vi "GUI_DS-LaserMachiningInputLogger.vi"() -> ()   [LabVIEW 2013]
uses:
  Shared/GUI_Template/GUI_master/tcp_new_data_event.ctl
  Shared/GUI_Template/GUI_master/tcp new data cluster.ctl
panel:
  out "tcp data event":T1
  in  "Refresh Button":bool
  out "XY Graph 4":cluster{timestamp[], dbl[]}(graph)
  in  "Boolean":bool=TRUE caption="Median filter"
  in  "Auto-scale horizontal range":bool caption="Force selected range"
  out "XY Graph 5":cluster{timestamp[], dbl[]}(graph)
  out "XY Graph 3":cluster{timestamp[], dbl[]}(graph)
  in  "Range graph3 (hours) 2":dbl=2.0 caption="Range (hours)"
  in  "MeanCounts::3":dbl caption="LM_Focuscam MeanCounts" min=0.0 max=999999999.0
  in  "MeanCounts::2":dbl caption="LM_Mirrorcam MeanCounts" min=0.0 max=999999999.0
  in  "MeanCounts::4":dbl caption="TS-253a_in MeanCounts" min=0.0 max=999999999.0
  in  "GUIdevice 4":string="TS-253a_in"
  in  "GUIdevice 3":string="LM_Focuscam"
  in  "GUIdevice 2":string="LM_Mirrorcam"
  in  "Number of hours in buffer":dbl=96.0
  out "Current array size":i32
  in  "Range \n(hours)":dbl=48.0
  out "XY Graph 2":cluster{timestamp[], dbl[]}(graph)
  in  "Range\n(hours)":dbl=2.0
  in  "refresh time (ms)":i32=2000
  out "XY Graph":cluster{timestamp[], dbl[]}(graph)
  in  "reading.var 1::1":dbl caption="Regen pulse energy" min=-100000.0 max=100000.0
  in  "stop":bool
  in  "GUIdevice 1":string="DS-LaserFrontEndLogger"
  # "Laser Machining Input logger"
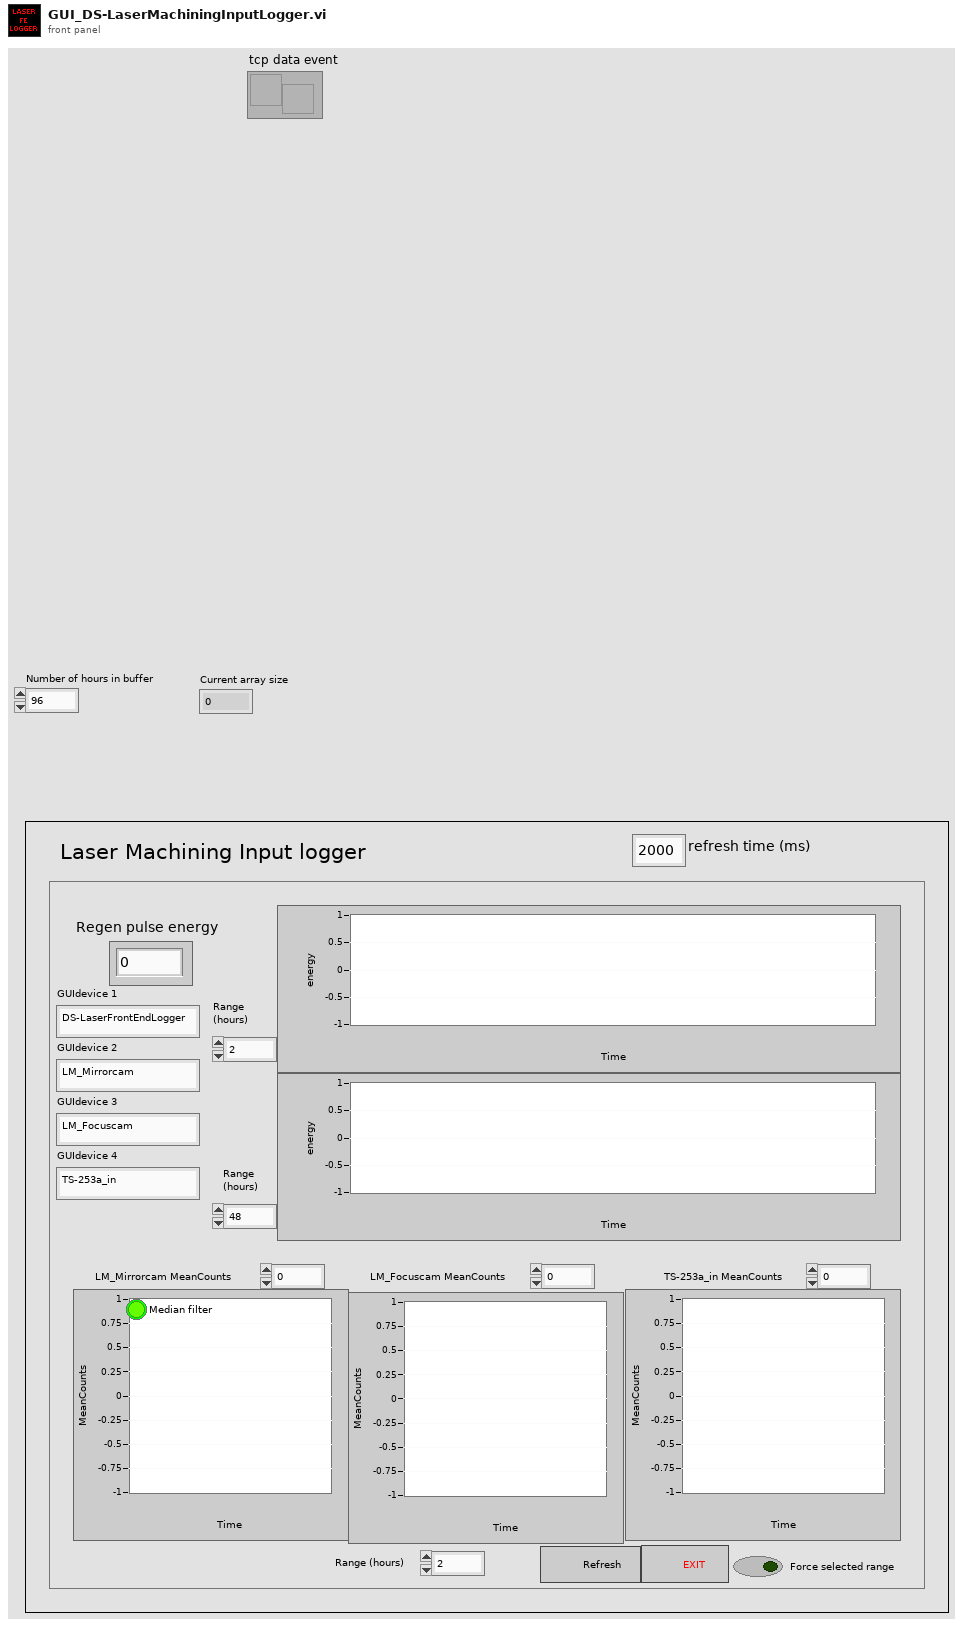
[diagram p1: front panel]
types:
  T1 = typedef "tcp_new_data_event.ctl" = refnum<user-event>
  T2 = enum32{"invalid app kind", "Development System", "Run Time System", "Student Edition", "Embedded LabVIEW", "Evaluation", "Custom"}
  T3 = typedef "tcp new data cluster.ctl" = cluster{"EventEnum":enum16{"new data", "connection status update"}, "Device name":string}
  T4 = enum32{"Invalid", "Standard", "Closed", "Hidden", "Minimized", "Maximized"}
  T5 = cluster{"Core":cluster{"Current VI Reference":refnum<vi>, "Close Panel on Exit?":bool}, "Your Boolean data":bool, "Your string data":string, "SuperGUI":cluster{"STOP queue":refnum<queue>, "SuperGUI ref":refnum<vi>}, "Data":cluster{"Timastamp":dbl[], "variable 1":dbl[], "variable 2":dbl[], "variable 3":dbl[], "variable 4":dbl[], "variable 5":dbl[]}}
  T6 = cluster{"Timastamp":dbl[], "variable 1":dbl[], "variable 2":dbl[], "variable 3":dbl[], "variable 4":dbl[], "variable 5":dbl[]}
  T7 = cluster{"STOP queue":refnum<queue>, "SuperGUI ref":refnum<vi>}
  T8 = cluster{"Current VI Reference":refnum<vi>, "Close Panel on Exit?":bool}
  T9 = cluster{"XY Graph":refnum<vi>, "XY Graph 2":refnum<vi>, "XY Graph 3":refnum<vi>, "XY Graph 4":refnum<vi>, "XY Graph 5":refnum<vi>}
  T10 = cluster{"XY graph":cluster{timestamp[], dbl[]}, "XY graph 2":cluster{timestamp[], dbl[]}, "XY graph 3":cluster{timestamp[], dbl[]}, "XY graph 4":cluster{timestamp[], dbl[]}, "XY graph 5":cluster{timestamp[], dbl[]}}
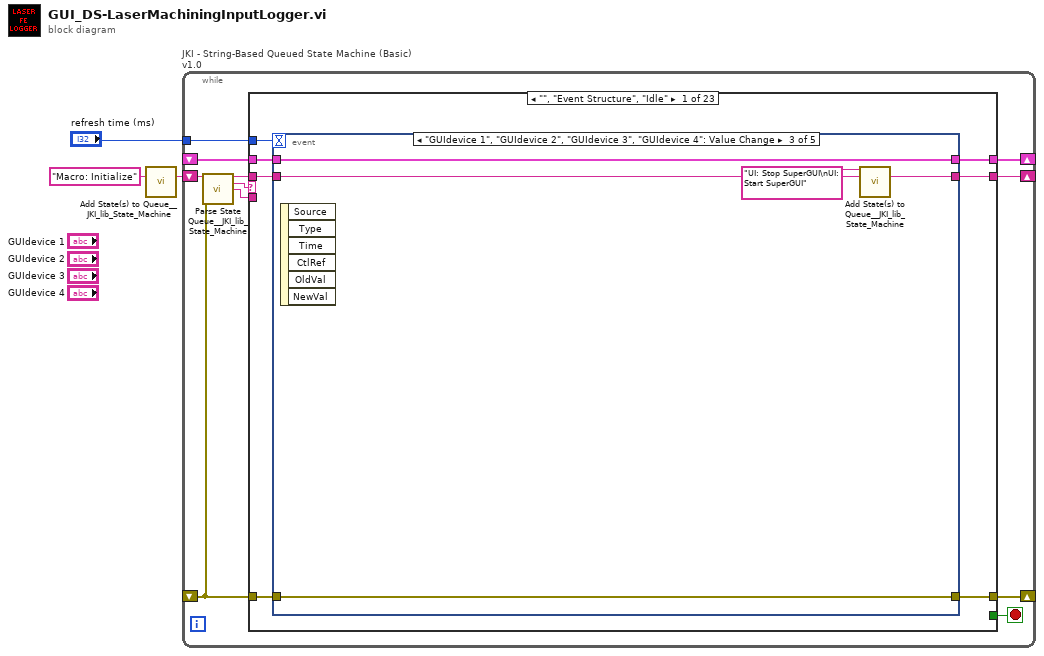
[diagram p0: block diagram]
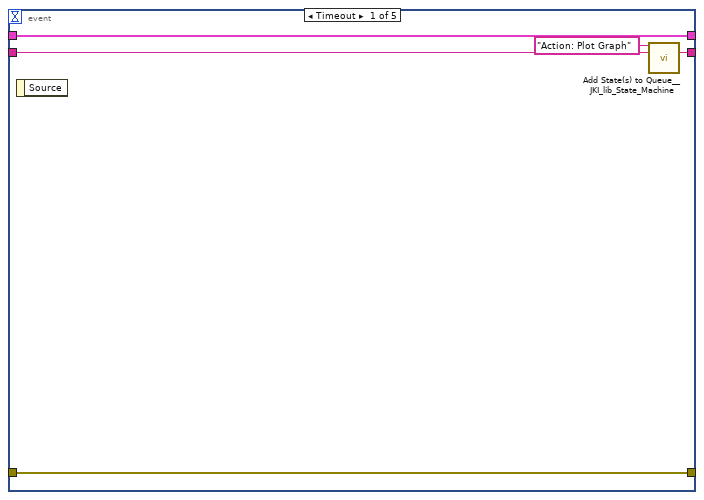
[diagram p2: hidden frame]
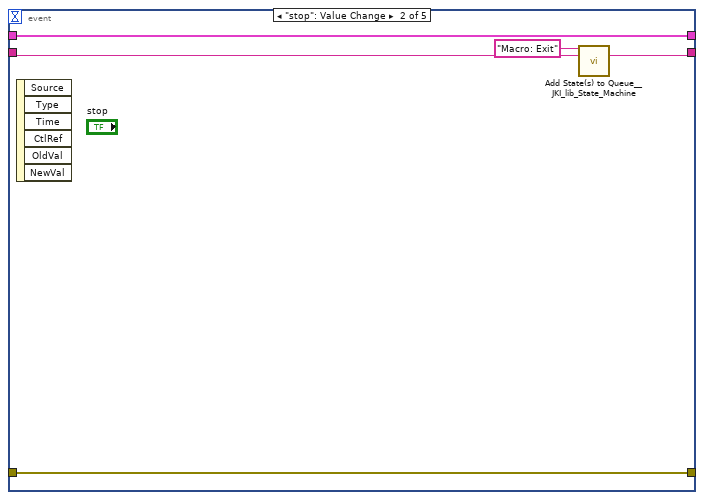
[diagram p3: hidden frame]
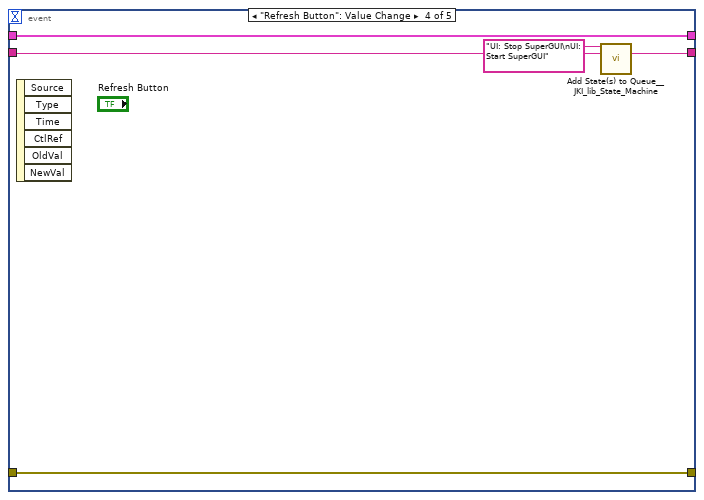
[diagram p4: hidden frame]
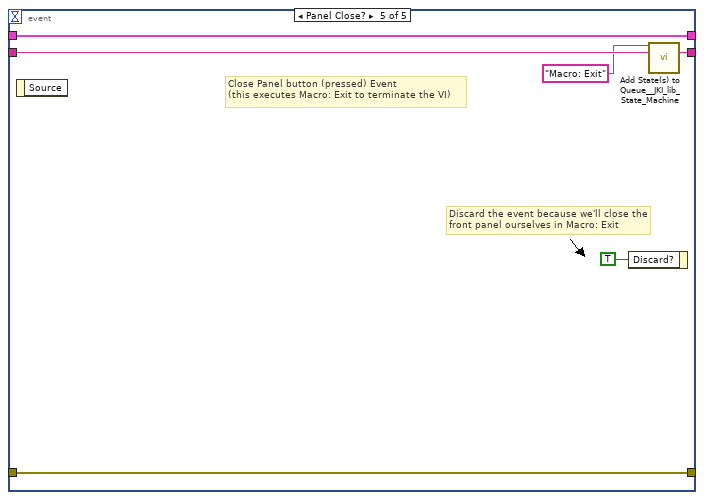
[diagram p5: hidden frame]
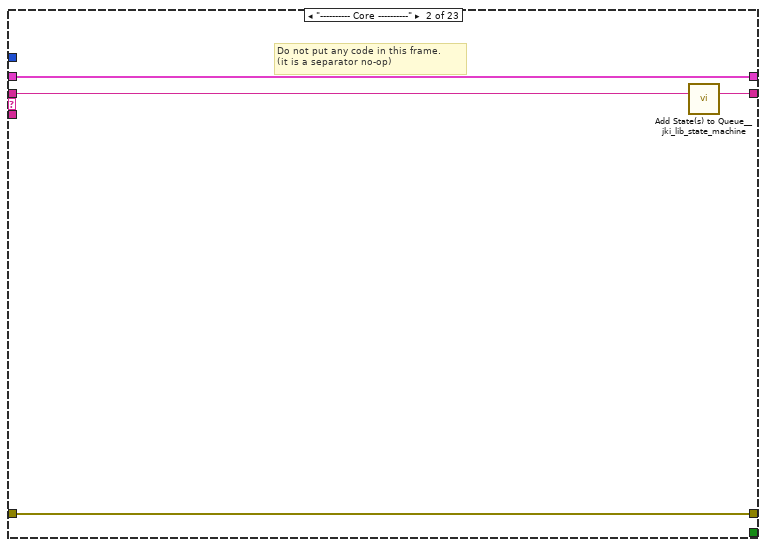
[diagram p6: hidden frame]
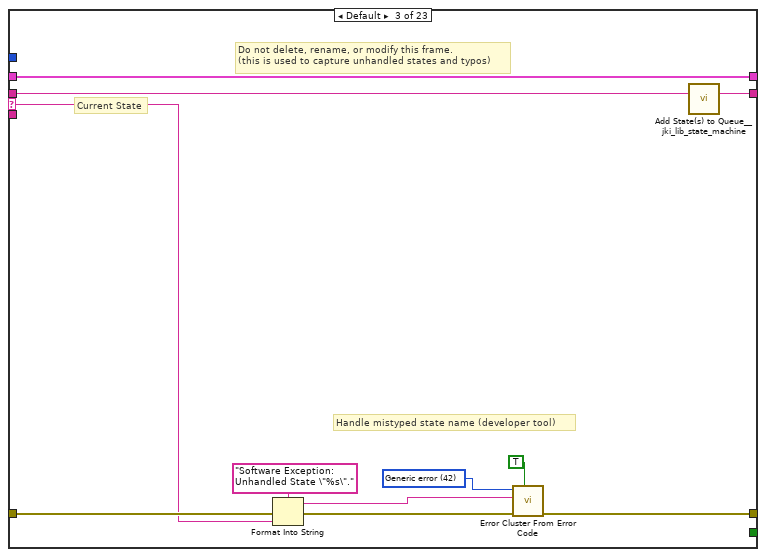
[diagram p7: hidden frame]
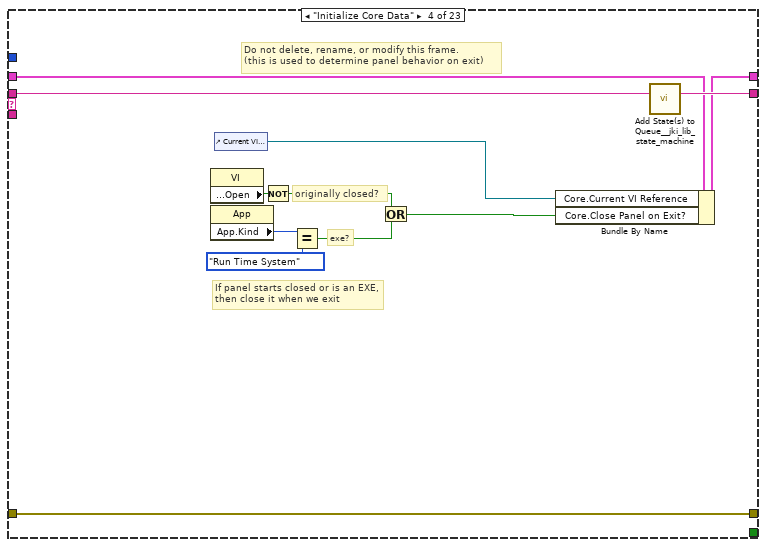
[diagram p8: hidden frame]
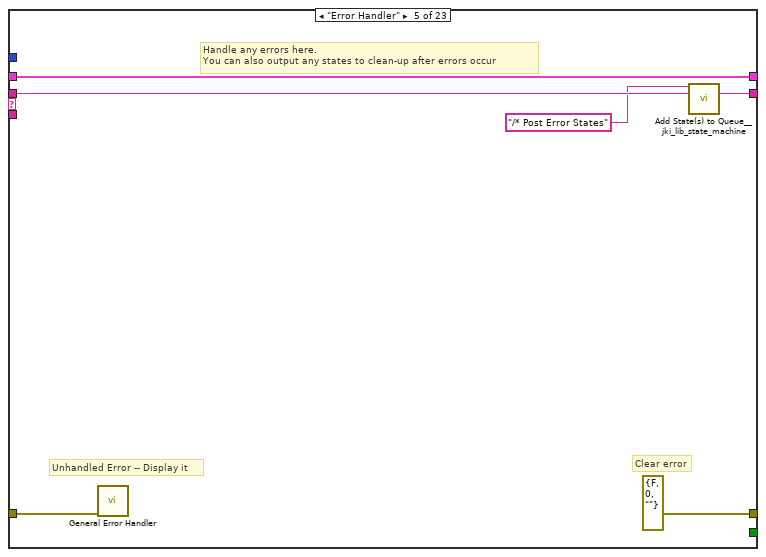
[diagram p9: hidden frame]
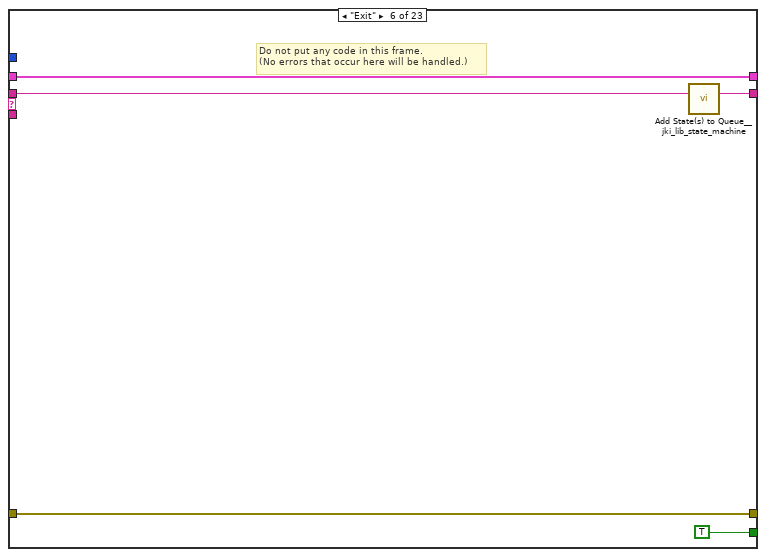
[diagram p10: hidden frame]
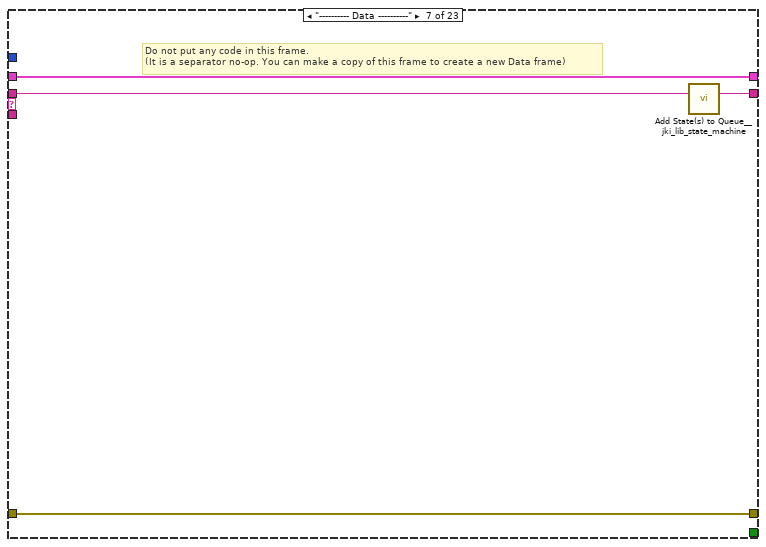
[diagram p11: hidden frame]
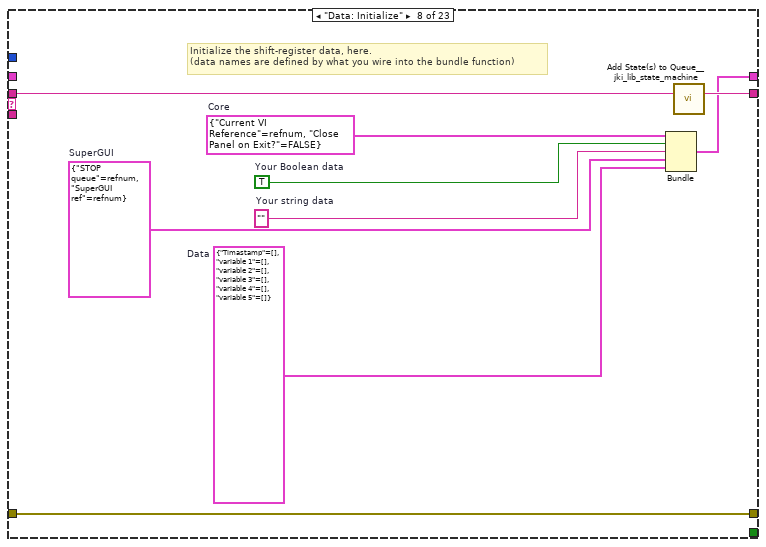
[diagram p12: hidden frame]
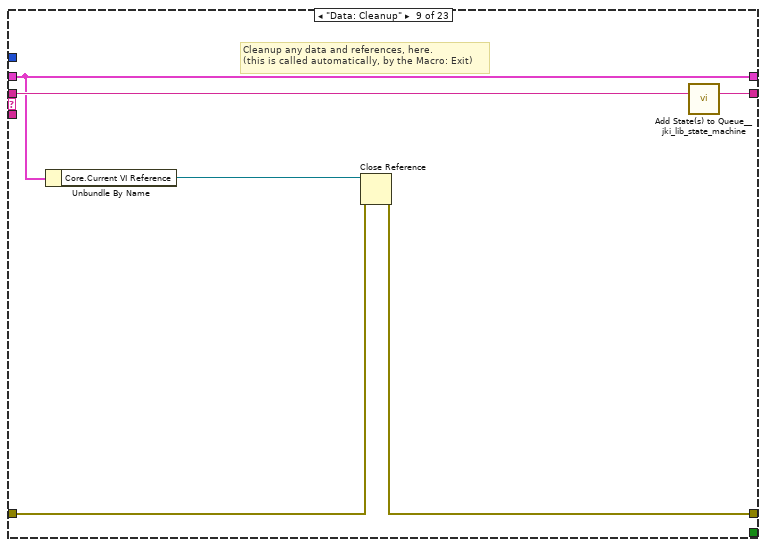
[diagram p13: hidden frame]
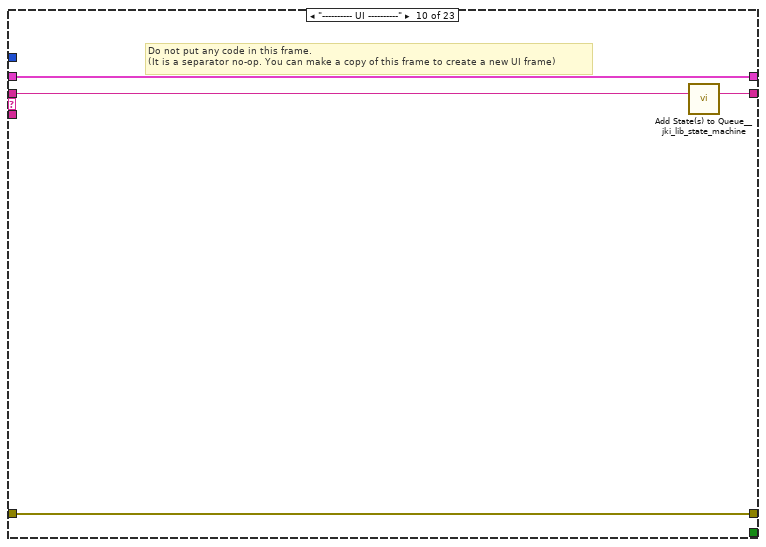
[diagram p14: hidden frame]
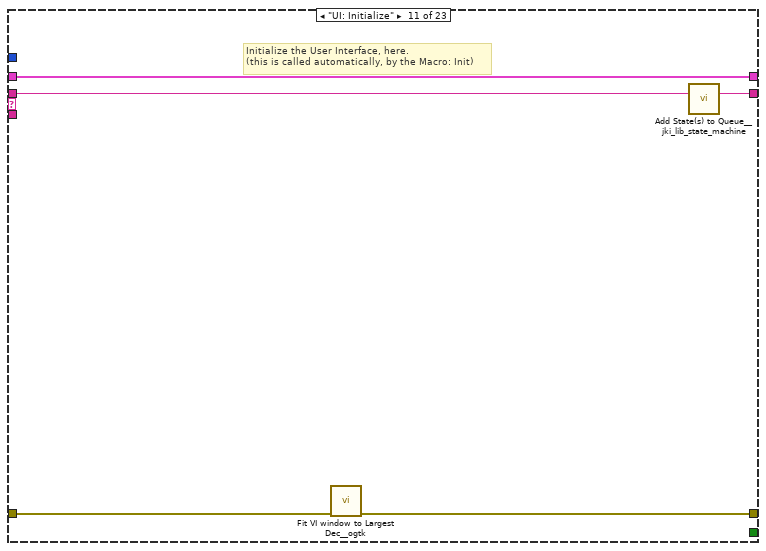
[diagram p15: hidden frame]
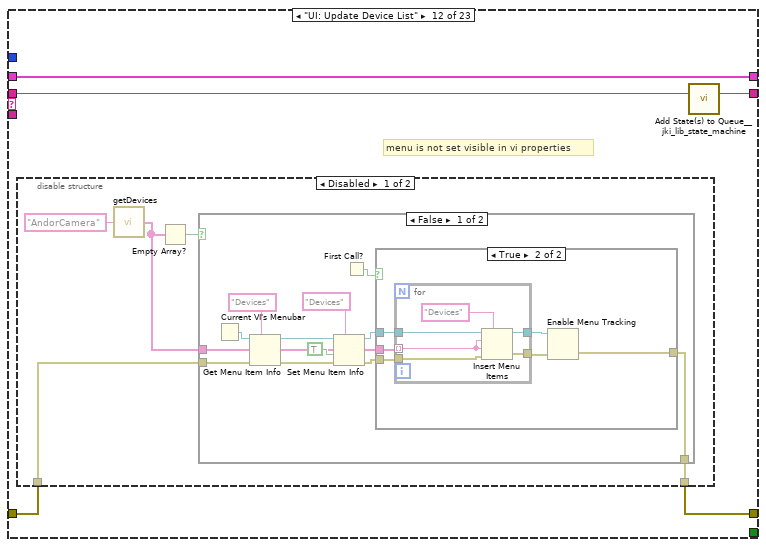
[diagram p16: hidden frame]
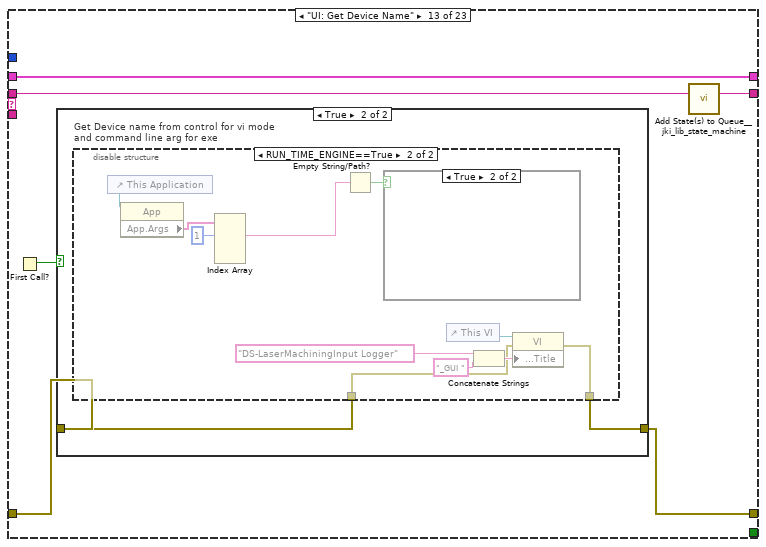
[diagram p20: hidden frame]
diagram:
  n1 = call <vilib>:"Add State(s) to Queue__JKI_lib_State_Machine.vi"("State(s) in (\"\")"="Macro: Initialize") -> ("States Out"=w3:string)  [unwired: 14 in]
  n2 = while "JKI - String-Based Queued State Machine (Basic) v1.0" {
    shift-right: [w7] -> _
    shift-left: _ -> [w6]
    shift-right: [w10] -> _
    shift-left: _ -> [w5]
    shift-right: [w9] -> _
    shift-left: w3 -> [w11]
    tunnel: "refresh time (ms)" -> [w4]
    stop <- w8 stop-if-true
    n3 = call <vilib>:"Parse State Queue__JKI_lib_State_Machine.vi"("State Queue"=w11, "Error In (no error)"=w5) -> ("Remaining States"=w13:string, "Current State"=w14:string, "Arguments"=w12:string)  [unwired: 11 in]
    n4 = case shown="\"\", \"Event Structure\", \"Idle\"" w14 {
      selector: w14 -> [_ _ w52 _ _ _ _ _ _ _ _ _ _ _ _ _ _ _ _ _ _ _ _]
      tunnel: w13 -> [w21 w51 w56 w74 w80 w85 w89 w98 w104 w108 w113 w118 w156 w190 w198 w204 w215 w241 w246 w256 w260 w293 w297]
      tunnel: w12 -> [_ _ _ _ _ _ _ _ _ _ _ _ _ _ _ w199 w209 _ _ _ _ _ _]
      tunnel: w6 -> [w19 w48 w54 w65 w77 w83 w86 _ w99 w105 w111 w116 w154 w181 w193 w202 w211 w238 w243 w253 w257 w269 w294]
      tunnel: [w18 w49 w58 w71 errorcluster {"status"=FALSE, "code"=0, "source"=""} ("error out") w82 w87 w95 w100 w106 w109 w114 w151 w174 w191 w200 w212 w239 w244 w254 w258 w291 w295] -> w10
      tunnel: w5 -> [w17 w49 w57 w71 w76 w82 w87 w95 w101 w106 w110 w115 w152 w175 w192 w201 w213 w239 w244 w254 w258 w291 w295]
      tunnel: [w20 w50 w55 w73 w79 w84 w88 w97 w103 w107 w112 w117 w155 w189 w197 w203 w214 w240 w245 w255 w259 w292 w296] -> w9
      tunnel: [_ _ _ _ _ TRUE _ _ _ _ _ _ _ _ _ _ _ _ _ _ _ _ _] -> w8
      tunnel: [w16 w48 w54 w72 w77 w83 w86 w96 w99 w105 w111 w116 w154 w180 w193 w202 w211 w238 w243 w253 w257 w268 w294] -> w7
      tunnel: w4 -> [w15 _ _ _ _ _ _ _ _ _ _ _ _ _ _ _ _ _ _ _ _ w283 _]
      frame "", "Event Structure", "Idle" {
        n5 = event shown="[2] \"GUIdevice 1\", \"GUIdevice 2\", \"GUIdevice 3\", \"GUIdevice 4\": Value Change" {
          selector: _ -> [_ _ _ _ _]
          dyn-events: _ -> [_ _ _ _ _]
          timeout: w15 -> [_ _ _ _ _]
          tunnel: w21 -> [w26 w29 w35 w39 w47]
          tunnel: [w25 w28 w34 w38 w46] -> w20
          tunnel: w19 -> [w23 w31 w36 w41 w44]
          tunnel: [w24 w30 w32 w40 w45] -> w18
          tunnel: w17 -> [w24 w30 w32 w40 w45]
          tunnel: [w23 w31 w36 w41 w44] -> w16
          event Timeout {
            n6 = event-data() -> ()  [unwired: 1 in, 1 out]
            n7 = call <vilib>:"Add State(s) to Queue__JKI_lib_State_Machine.vi"("State(s) in Front (\"\")"="Action: Plot Graph" ("State(s) in Front (\"\")"), "State(s) in (\"\")"=w26) -> ("States Out"=w25:string)  [unwired: 13 in]
          }
          event "stop": Value Change {
            n8 = event-data() -> ()  [unwired: 1 in, 6 out]
            n9 = call <vilib>:"Add State(s) to Queue__JKI_lib_State_Machine.vi"("State(s) in Front (\"\")"="Macro: Exit", "State(s) in (\"\")"=w29) -> ("States Out"=w28:string)  [unwired: 13 in]
          }
          event "GUIdevice 1", "GUIdevice 2", "GUIdevice 3", "GUIdevice 4": Value Change {
            n10 = event-data() -> ()  [unwired: 1 in, 6 out]
            n11 = call <vilib>:"Add State(s) to Queue__JKI_lib_State_Machine.vi"("State(s) in Front (\"\")"="UI: Stop SuperGUI\nUI: Start SuperGUI", "State(s) in (\"\")"=w35) -> ("States Out"=w34:string)  [unwired: 13 in]
          }
          event "Refresh Button": Value Change {
            n12 = event-data() -> ()  [unwired: 1 in, 6 out]
            n13 = call <vilib>:"Add State(s) to Queue__JKI_lib_State_Machine.vi"("State(s) in Front (\"\")"="UI: Stop SuperGUI\nUI: Start SuperGUI", "State(s) in (\"\")"=w39) -> ("States Out"=w38:string)  [unwired: 13 in]
          }
          event Panel Close? {
            # "Discard the event because we'll close the front panel ourselves in Macro: Exit"
            # "Close Panel button (pressed) Event\n(this executes Macro: Exit to terminate the VI)"
            n14 = event-data() -> ()  [unwired: 1 in, 1 out]
            n15 = event-data("Discard?"=TRUE) -> ()  [unwired: 1 in, 1 out]
            n16 = call <vilib>:"Add State(s) to Queue__JKI_lib_State_Machine.vi"("State(s) in Front (\"\")"="Macro: Exit", "State(s) in (\"\")"=w47) -> ("States Out"=w46:string)  [unwired: 13 in]
          }
        }
      }
      frame "---------- Core ----------" {
        # "Do not put any code in this frame.\n(it is a separator no-op)"
        n17 = call <vilib>:"Add State(s) to Queue__jki_lib_state_machine.vi"("State(s) in (\"\")"=w51) -> ("States Out"=w50:string)  [unwired: 14 in]
      }
      frame Default {
        w61 = 42 items=["No error", "Argument error", "Memory is full", "Out of zone", "End of file", "File already open", "Generic file I/O error", "File not found", "File permission error", "Disk is full", "Duplicate path", "Too many files open", "System feature not enabled", "Resource file not found", "Cannot add resource", "Resource not found", "Image not found", "Image memory error", "Pen does not exist", "Config type invalid", "Config token not found", "Config parse error", "Config memory error", "Bad external code format", "Bad external code offset", "External code not present", "Null window", "Destroy window error", "Null menu", "Print aborted", "Bad print record", "Print driver error", "Windows error during printing", "Memory error during printing", "Print dialog error", "Generic print error", "Invalid device refnum", "Device not found", "Device parameter error", "Device unit error", "Cannot open device", "Device call aborted", "Generic error", "Cancelled by user", "Object ID too low", "Object ID too high", "Object not in heap", "Unknown heap", "Unknown object (invalid DefProc)", "Unknown object (DefProc not in table)", "Message out of range", "Invalid (null) method", "Unknown message", "Manager call not supported", "Bad address", "Network operation in progress", "Network operation timed out", "Connection is busy", "Network attribute not supported", "Network error", "Address in use", "System out of memory", "Connection aborted", "Connection refused", "Not connected", "Already connected", "Connection closed", "Initialization error (interapplication manager)", "Bad occurrence", "Wait on unbound occurrence handler", "Occurrence queue overflow", "Datalog type conflict", "Unused", "Unrecognized type (interapplication manager)", "Memory corrupt", "Failed to make temporary DLL", "Old CIN version", "Drag socket not found", "Failed to load drop-object", "Failed to register OLE object", "Failed to release OLE object", "Format specifier type mismatch", "Unknown format specifier", "Too few format specifiers", "Too many format specifiers", "Scan failed", "Newer CIN version", "Error converting to variant", "Runtime menu error", "Password tampered", "Variant attribute not found", "Incompatible variant data type", "Event data is not available", "Event Store is not present", "Occurrence is not found", "Event Queue is not created", "Event info is not available", "Refnum passed is NULL", "Error retrieving Class GUID", "Error retrieving CoClass GUID", "Error retrieving TypeLib GUID.", "Bad built application magic bytes.", "Specific driver is different from the specific driver associated with the Logical Name.", "There is no session opened to the class driver.", "Max Error", "MAX - Error with config objects", "MAX - Error loading configuration", "MAX - Group not supported"]
        # "Current State"
        # "Do not delete, rename, or modify this frame.\n(this is used to capture unhandled states and typos)"
        # "Handle mistyped state name (developer tool)"
        n18 = Format Into String(format string="Software Exception: Unhandled State \"%s\"." ("message"), error in=w57, w52) -> (resulting string=w60:string, error out=w59:errorcluster)  [unwired: 1 in]
        n19 = call <vilib>:"Error Cluster From Error Code.vi"("show call chain? (False)"=TRUE, "error in (no error)"=w59, "error message (\"\")"=w60, "error code (0)"=w61) -> ("error out"=w58:errorcluster)  [unwired: 5 in]
        n20 = call <vilib>:"Add State(s) to Queue__jki_lib_state_machine.vi"("State(s) in (\"\")"=w56) -> ("States Out"=w55:string)  [unwired: 14 in]
      }
      frame "Initialize Core Data" {
        # "Do not delete, rename, or modify this frame.\n(this is used to determine panel behavior on exit)"
        # "originally closed?"
        # "exe?"
        # "If panel starts closed or is an EXE, then close it when we exit"
        n21 = property class="VI"() -> ("Front Panel.Open"=w70:bool)  [unwired: 2 in, 2 out]
        n22 = property class="App"() -> ("App.Kind"=w69:T2)  [unwired: 2 in, 2 out]
        n23 = control-ref of="Current VI Reference"() -> (w63:refnum<vi>)
        n24 = Not(x=w70) -> (.not. x?=w67:bool)
        n25 = Equal?(x=w69, y=T2."Run Time System" ("Application:Kind")) -> (x = y?=w66:bool)
        n26 = Or(x=w67, y=w66) -> (x .or. y?=w64:bool)
        n27 = Bundle By Name(cluster=w65, "Core.Current VI Reference"=w63, "Core.Close Panel on Exit?"=w64) -> (w72:T5)
        n28 = call <vilib>:"Add State(s) to Queue__jki_lib_state_machine.vi"("State(s) in (\"\")"=w74) -> ("States Out"=w73:string)  [unwired: 14 in]
      }
      frame "Error Handler" {
        # "Unhandled Error -- Display it"
        # "Handle any errors here.\nYou can also output any states to clean-up after errors occur"
        # "Clear error"
        n29 = call <vilib>:"General Error Handler.vi"("error in (no error)"=w76) -> ()  [unwired: 10 in, 5 out]
        n30 = call <vilib>:"Add State(s) to Queue__jki_lib_state_machine.vi"("State(s) in Front (\"\")"="/* Post Error States", "State(s) in (\"\")"=w80) -> ("States Out"=w79:string)  [unwired: 13 in]
      }
      frame "Exit" {
        # "Do not put any code in this frame.\n(No errors that occur here will be handled.)"
        n31 = call <vilib>:"Add State(s) to Queue__jki_lib_state_machine.vi"("State(s) in (\"\")"=w85) -> ("States Out"=w84:string)  [unwired: 14 in]
      }
      frame "---------- Data ----------" {
        # "Do not put any code in this frame.\n(It is a separator no-op. You can make a copy of this frame to create a new Data frame)"
        n32 = call <vilib>:"Add State(s) to Queue__jki_lib_state_machine.vi"("State(s) in (\"\")"=w89) -> ("States Out"=w88:string)  [unwired: 14 in]
      }
      frame "Data: Initialize" {
        w90 = T6 {"Timastamp"=[], "variable 1"=[], "variable 2"=[], "variable 3"=[], "variable 4"=[], "variable 5"=[]}  # Data
        w91 = T7 {"STOP queue"=refnum, "SuperGUI ref"=refnum}  # SuperGUI
        w92 = T8 {"Current VI Reference"=refnum, "Close Panel on Exit?"=FALSE}  # Core
        w94 = TRUE  # Your Boolean data
        w93 = ""  # Your string data
        # "Initialize the shift-register data, here.\n(data names are defined by what you wire into the bundle function)"
        n33 = Bundle("Core"=w92, "Your Boolean data"=w94, "Your string data"=w93, "SuperGUI"=w91, "Data"=w90) -> (w96:T5)  [unwired: 1 in]
        n34 = call <vilib>:"Add State(s) to Queue__jki_lib_state_machine.vi"("State(s) in (\"\")"=w98) -> ("States Out"=w97:string)  [unwired: 14 in]
      }
      frame "Data: Cleanup" {
        # "Cleanup any data and references, here.\n(this is called automatically, by the Macro: Exit)"
        n35 = Unbundle By Name(w99) -> ("Core.Current VI Reference"=w102:refnum<vi>)
        n36 = Close Reference(reference=w102, error in (no error)=w101) -> (error out=w100:errorcluster)
        n37 = call <vilib>:"Add State(s) to Queue__jki_lib_state_machine.vi"("State(s) in (\"\")"=w104) -> ("States Out"=w103:string)  [unwired: 14 in]
      }
      frame "---------- UI ----------" {
        # "Do not put any code in this frame.\n(It is a separator no-op. You can make a copy of this frame to create a new UI frame)"
        n38 = call <vilib>:"Add State(s) to Queue__jki_lib_state_machine.vi"("State(s) in (\"\")"=w108) -> ("States Out"=w107:string)  [unwired: 14 in]
      }
      frame "UI: Initialize" {
        # "Initialize the User Interface, here.\n(this is called automatically, by the Macro: Init)"
        n39 = call <userlib>:"Fit VI window to Largest Dec__ogtk.vi"("error in (no error)"=w110) -> ("error out"=w109:errorcluster)  [unwired: 5 in, 1 out]
        n40 = call <vilib>:"Add State(s) to Queue__jki_lib_state_machine.vi"("State(s) in (\"\")"=w113) -> ("States Out"=w112:string)  [unwired: 14 in]
      }
      frame "UI: Update Device List" {
        # "menu is not set visible in vi properties"
        n41 = disable-structure shown="Disabled" {
          disable-tunnel: w115 -> [w123 w150]
          disable-tunnel: [w121 w150] -> w114
          frame Disabled {
            n42 = call "getDevices.vi"("Device Class"="AndorCamera") -> ("All Devices"=w119:string[])
            n43 = Empty Array?(array=w119) -> (empty?=w120:bool)
            n44 = case shown="False" w120 {
              tunnel: w123 -> [w126 w149]
              tunnel: [w125 w149] -> w121
              tunnel: w119 -> [w124 _]
              frame False {
                n45 = Current VI's Menubar() -> (w129:refnum<k9>)
                n46 = Get Menu Item Info(7:"Devices" ("item tag"), 8:w126, 11:w129) -> (0:w135:errorcluster, 3:w131:refnum<k9>)  [unwired: 5 out]
                n47 = Set Menu Item Info(7:"Devices" ("item tag"), 8:w135, 9:TRUE ("enabled"), 11:w131) -> (0:w134:errorcluster, 3:w133:refnum<k9>)  [unwired: 3 in]
                n48 = First Call?() -> (First Call?: T/F=w127:bool)
                n49 = case shown="True" w127 {
                  tunnel: w133 -> [_ w141]
                  tunnel: w124 -> [_ w140]
                  tunnel: w134 -> [w136 w138]
                  tunnel: [w136 w137] -> w125
                  frame False {
                  }
                  frame True {
                    n50 = for {
                      tunnel: [w148] -> w142
                      tunnel: w140 -> [w146] mode=indexing
                      tunnel: w141 -> [w145]
                      tunnel: [w144] -> w139
                      tunnel: w138 -> [w143]
                      n51 = Insert Menu Items(5:"Devices" ("menu tag"), 6:w143, 7:w146, 8:w146, 9:w145) -> (0:w144:errorcluster, 3:w148:refnum<k9>)  [unwired: 1 in, 1 out]
                    }
                    n52 = Enable Menu Tracking(2:w139, 4:w142) -> (0:w137:errorcluster)  [unwired: 1 in, 1 out]
                  }
                }
              }
              frame True {
              }
            }
          }
          frame Enabled {
          }
        }
        n53 = call <vilib>:"Add State(s) to Queue__jki_lib_state_machine.vi"("State(s) in (\"\")"=w118) -> ("States Out"=w117:string)  [unwired: 14 in]
      }
      frame "UI: Get Device Name" {
        n54 = First Call?() -> (First Call?: T/F=w153:bool)
        n55 = case shown="True" w153 {
          tunnel: w152 -> [w157 w159]
          tunnel: [w157 w158] -> w151
          frame False {
          }
          frame True {
            n56 = disable-structure "Get Device name from control for vi mode\nand command line arg for exe" shown="RUN_TIME_ENGINE==True" {
              disable-tunnel: w159 -> [_ w163]
              disable-tunnel: [_ w162] -> w158
              frame condition #0 (active) {
              }
              frame condition #1 {
                n57 = control-ref of="This Application"() -> (w170:refnum<vi>)
                n58 = property class="App"(reference=w170) -> ("App.Args"=w169:string[])  [unwired: 1 in, 2 out]
                n59 = Index Array(array=w169, index #1=1 ("index")) -> (element #1=w161:string)  [unwired: 3 in, 3 out]
                n60 = Empty String/Path?(string/path=w161) -> (empty?=w167:bool)
                n61 = case shown="True" w167 {
                  frame False {
                  }
                  frame True {
                  }
                }
                n62 = control-ref of="This VI"() -> (w166:refnum<vi>)
                n63 = Concatenate Strings("DS-LaserMachiningInput Logger" ("string"), "_GUI ") -> (w165:string)
                n64 = property class="VI"(reference=w166, error in=w163, "Front Panel.Title"=w165) -> (error out=w162:errorcluster)  [unwired: 1 out]
              }
            }
          }
        }
        n65 = call <vilib>:"Add State(s) to Queue__jki_lib_state_machine.vi"("State(s) in (\"\")"=w156) -> ("States Out"=w155:string)  [unwired: 14 in]
      }
      frame "UI: Start SuperGUI" {
        # "create stop queue for supergui and its clones"
        # "x100 abort will be dependent on caller VI\nx80 abort will be independent of caller vi, this will abort vi when labview is closed."
        # "Start SuperGUI asynchronous way"
        n66 = vi-ref "GUI_Master_subvi_reentrant_queues.vi"() -> (w173:refnum<vi>)
        n67 = property class="VI"(reference=w173) -> ("Path"=w172:path)  [unwired: 1 in, 2 out]
        n68 = Create User Event(user event datatype=T3 {"EventEnum"=enum."new data", "Device name"="Device name"} ("New Event"), error in=w175) -> (user event=w176:refnum<user-event>, error out=w182:errorcluster)
        "tcp data event" <- w176
        n69 = control-ref of="This Application"() -> (w179:refnum<vi>)
        n70 = control-ref of="This VI"() -> (w178:refnum<vi>)
        n71 = Open VI Reference(type specifier VI Refnum (for type only)=refnum<vi> refnum, vi path=w172, options=256) -> (vi reference=w188:refnum<vi>, error out=w187:errorcluster)  [unwired: 3 in]
        n72 = register-events(w176) -> ()  [unwired: 2 in, 2 out]
        n73 = call "supergui create stop queue.vi"() -> ("STOP Queue out"=w184:refnum<queue>)  [unwired: 11 in]
        n74 = Current VI's Menubar() -> (w177:refnum<k9>)
        n75 = call-by-ref "Start Asynchronous Call"(reference=w188, error in=w187, "STOP Queue in"=w184, "This Application"=w179, 8:"error in (no error)"=w182, "tcp data event"=w176, "Caller menu reference"=w177, "Caller VI ref"=w178) -> (reference out=w171:refnum<vi>, error out=w174:errorcluster)  [unwired: 5 in, 1 out]
        n76 = Bundle By Name(cluster=w181, "SuperGUI.SuperGUI ref"=w171, "SuperGUI.STOP queue"=w184) -> (w180:T5)
        n77 = call <vilib>:"Add State(s) to Queue__jki_lib_state_machine.vi"("State(s) in (\"\")"=w190) -> ("States Out"=w189:string)  [unwired: 14 in]
      }
      frame "UI: Stop SuperGUI" {
        # "Stop Supergui Clone and wait until it exit properly"
        n78 = Unbundle By Name(w193) -> ("SuperGUI.SuperGUI ref"=w195:refnum<vi>, "SuperGUI.STOP queue"=w194:refnum<queue>)
        n79 = Release Queue(queue=w194, error in (no error)=w192) -> (error out=w196:errorcluster)  [unwired: 1 in, 2 out]
        n80 = call-by-ref "Wait On Asynchronous Call"(reference=w195, error in=w196) -> ("error out"=w191:errorcluster)  [unwired: 11 in, 2 out]
        n81 = call <vilib>:"Add State(s) to Queue__jki_lib_state_machine.vi"("State(s) in (\"\")"=w198) -> ("States Out"=w197:string)  [unwired: 14 in]
      }
      frame "UI: Cursor Set" {
        # "Argument"
        # "Set and Unset Cursor Busy.\n(Usage: \"UI: Cursor Set >> Busy|Idle\")"
        n82 = case shown="\"Idle\", Default" w199 {
          tunnel: w201 -> [w206 w208]
          tunnel: [w205 w207] -> w200
          frame "Idle", Default {
            n83 = call <vilib>:"Unset Busy.vi"("error in (no error)"=w206) -> ("error out"=w205:errorcluster)  [unwired: 10 in]
          }
          frame "Busy" {
            n84 = call <vilib>:"Set Busy.vi"("error in (no error)"=w208) -> ("error out"=w207:errorcluster)  [unwired: 9 in, 1 out]
          }
        }
        n85 = call <vilib>:"Add State(s) to Queue__jki_lib_state_machine.vi"("State(s) in (\"\")"=w204) -> ("States Out"=w203:string)  [unwired: 14 in]
      }
      frame "UI: Front Panel State" {
        # "Argument"
        # "Set Front Panel Open or Closed\n(Usage: \"UI: Front Panel State >> Open|Close\")"
        n86 = Unbundle By Name(w211) -> ("Core.Current VI Reference"=w210:refnum<vi>)
        n87 = case shown="\"Close\"" w209 {
          tunnel: w213 -> [w219 w232]
          tunnel: [w221 w233] -> w212
          tunnel: w210 -> [w220 w230]
          frame "Open", Default {
            n88 = property class="VI"(reference=w220, error in=w219) -> (reference out=w217:refnum<vi>, error out=w218:errorcluster, "Front Panel.Open"=w216:bool)
            n89 = case shown="False" w216 {
              tunnel: [w224 w227] -> w221
              tunnel: w218 -> [w223 w227]
              tunnel: w217 -> [w222 _]
              frame False {
                n90 = invoke class="VI" method="FP.Open"(reference=w222, error in=w223, "Activate"=TRUE, "State"=T4."Standard") -> (error out=w224:errorcluster)  [unwired: 1 in, 4 out]
              }
              frame True {
              }
            }
          }
          frame "Close" {
            n91 = property class="VI"(reference=w230, error in=w232) -> (reference out=w229:refnum<vi>, error out=w231:errorcluster, "Front Panel.Open"=w228:bool)
            n92 = case shown="True" w228 {
              tunnel: [w234 w237] -> w233
              tunnel: w231 -> [w234 w236]
              tunnel: w229 -> [_ w235]
              frame False {
              }
              frame True {
                n93 = invoke class="VI" method="FP.Close"(reference=w235, error in=w236) -> (error out=w237:errorcluster)  [unwired: 1 in, 2 out]
              }
            }
          }
        }
        n94 = call <vilib>:"Add State(s) to Queue__jki_lib_state_machine.vi"("State(s) in (\"\")"=w215) -> ("States Out"=w214:string)  [unwired: 14 in]
      }
      frame "---------- Macro ----------" {
        # "Do not put any code in this frame.\n(It is a separator no-op. You can make a copy of this frame to create a new Macro frame)"
        n95 = call <vilib>:"Add State(s) to Queue__jki_lib_state_machine.vi"("State(s) in (\"\")"=w241) -> ("States Out"=w240:string)  [unwired: 14 in]
      }
      frame "Macro: Initialize" {
        # "Initialization Macro\n(This is called once, when the VI starts)"
        n96 = call <vilib>:"Add State(s) to Queue__jki_lib_state_machine.vi"("State(s) in Front (\"\")"="Data: Initialize\nInitialize Core Data\nUI: Initialize\nUI: Update Device List\nUI: Get Device Name\nUI: Start SuperGUI\nUI: Front Panel State >> Open", "State(s) in (\"\")"=w246) -> ("States Out"=w245:string)  [unwired: 13 in]
      }
      frame "Macro: Exit" {
        # "Exit Macro\n(This is called once, when the VI exits)"
        n97 = Unbundle By Name(w253) -> ("Core.Close Panel on Exit?"=w252:bool)
        n98 = Select(t="UI: Front Panel State >> Close", s=w252, f="") -> (s? t:f=w249:string)
        n99 = call <vilib>:"Add State(s) to Queue__jki_lib_state_machine.vi"("State(s) in (\"\")"=w249, "State(s) at Back (\"\")"="Data: Cleanup\nExit") -> ("States Out"=w247:string)  [unwired: 13 in]
        n100 = call <vilib>:"Add State(s) to Queue__jki_lib_state_machine.vi"("State(s) in Front (\"\")"=w247, "State(s) in (\"\")"=w256) -> ("States Out"=w255:string)  [unwired: 13 in]
      }
      frame "---------- New Category ----------" {
        # "Template Separator\n(You can make a copy of, or modify, this frame)"
        n101 = call <vilib>:"Add State(s) to Queue__jki_lib_state_machine.vi"("State(s) in (\"\")"=w260) -> ("States Out"=w259:string)  [unwired: 14 in]
      }
      frame "Action: Plot Graph" {
        (unwired) T6 {"Timastamp"=[], "variable 1"=[], "variable 2"=[], "variable 3"=[], "variable 4"=[], "variable 5"=[]}  # Data
        w276 = T9 {"XY Graph"=refnum, "XY Graph 2"=refnum, "XY Graph 3"=refnum, "XY Graph 4"=refnum, "XY Graph 5"=refnum}  # Graph ref
        n102 = Unbundle By Name(w269) -> ("Data"=w284:T6)
        n103 = call "Get Graph Data.vi"("refresh time (ms)"=w283, "reading.var 1::1"="reading.var 1::1", "Number of hours in buffer"="Number of hours in buffer", "MeanCounts::2"="MeanCounts::2", "MeanCounts::3"="MeanCounts::3", "MeanCounts::4"="MeanCounts::4", "Data ip"=w284) -> ("Data op"=w277:T6, "Current array size"=→"Current array size":i32)  [unwired: 11 in]
        n104 = control-ref of="XY Graph"() -> (w275:refnum<vi>)
        n105 = control-ref of="XY Graph 2"() -> (w274:refnum<vi>)
        n106 = control-ref of="XY Graph 3"() -> (w273:refnum<vi>)
        n107 = control-ref of="XY Graph 4"() -> (w272:refnum<vi>)
        n108 = control-ref of="XY Graph 5"() -> (w271:refnum<vi>)
        n109 = Bundle By Name(cluster=w276, "XY Graph"=w275, "XY Graph 2"=w274, "XY Graph 3"=w273, "XY Graph 4"=w272, "XY Graph 5"=w271) -> (w270:T9)
        n110 = call "Display graph.vi"("Data ip"=w277, "Graph reference"=w270, "Range (hours)"="Range\n(hours)", "Range (hours) 2"="Range graph3 (hours) 2", "Range graph3 (hours) in"="Range \n(hours)", "Boolean"="Boolean", "Auto-scale \nhorizontal range"="Auto-scale horizontal range") -> ("Data op"=w267:T6, "XY graph"=w266:T10)  [unwired: 7 in]
        n111 = Unbundle By Name(w266) -> ("XY graph"=→"XY Graph":cluster{timestamp[], dbl[]}, "XY graph 2"=→"XY Graph 2":cluster{timestamp[], dbl[]}, "XY graph 3"=→"XY Graph 3":cluster{timestamp[], dbl[]}, "XY graph 4"=→"XY Graph 4":cluster{timestamp[], dbl[]}, "XY graph 5"=→"XY Graph 5":cluster{timestamp[], dbl[]})
        n112 = Bundle By Name(cluster=w269, "Data"=w267) -> (w268:T5)
        n113 = call <vilib>:"Add State(s) to Queue__jki_lib_state_machine.vi"("State(s) in (\"\")"=w293) -> ("States Out"=w292:string)  [unwired: 14 in]
      }
      frame "New Category: 2" {
        # "Your code here.\n(You can make a copy of, or modify, this frame)"
        n114 = call <vilib>:"Add State(s) to Queue__jki_lib_state_machine.vi"("State(s) in (\"\")"=w297) -> ("States Out"=w296:string)  [unwired: 14 in]
      }
    }
  }
